vi "Single motor operation(Wheel mode).vi"() -> ()   [LabVIEW 2016]
uses:
  <instrlib>/Dynamixel Motor/Public/Motor Operation/Low Level/Baud Setting.ctl
  <instrlib>/Dynamixel Motor/Dynamixel Motor.lvlib
panel:
  in  "Goal Speed (RPM)":dbl
  in  "Motor ID (0)":u8
  in  "정지":bool
  in  "Baud rate (57600 bps)":T1=34 items=["1,000,000 bps"=1, "500,000 bps"=3, "400,000 bps"=4, "250,000 bps"=7, "200,000 bps"=9, "115200 bps"=16, "57600 bps"=34, "19200 bps"=103, "9600 bps"=207]
  in  "VISA resource name":refnum<visa-resource-name>
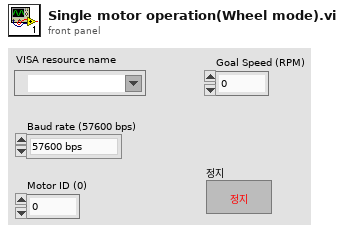
[diagram p1: front panel]
types:
  T1 = typedef "Dynamixel Motor.lvlib/Baud Setting.ctl" = u8
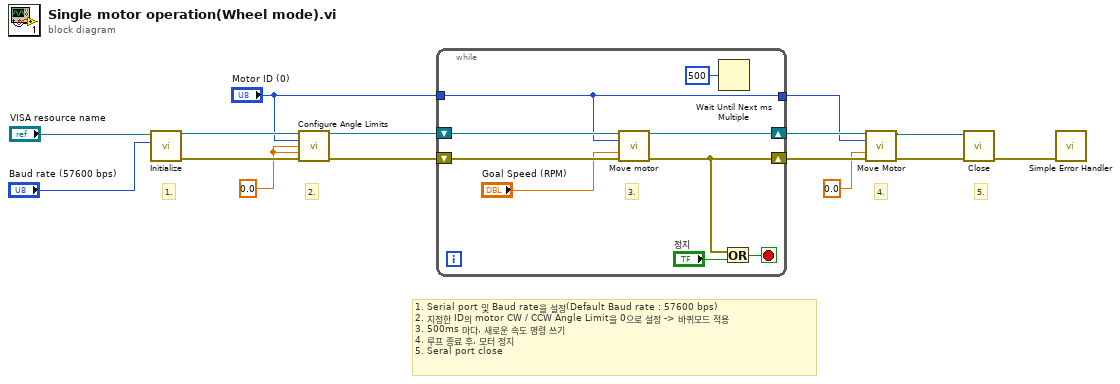
[diagram p0: block diagram]
diagram:
  w8 = 0.0 ("Clockwise Angle Limit (0 deg)")
  # "5."
  # "1. Serial port 및 Baud rate을 설정(Default Baud rate : 57600 bps)\n2. 지정한 ID의 motor CW / CCW Angle Limit을 0으로 설정 -> 바퀴모드 적용\n3. 500ms 마다, 새로운 속도 명령 쓰기\n4. 루프 종료 후, 모터 정지\n5. Seral port close"
  # "2."
  # "4."
  # "1."
  n1 = call <instrlib>:"Initialize.vi"("Baud rate (57600 bps)"="Baud rate (57600 bps)", "VISA resource name"="VISA resource name") -> ("error out"=w14:errorcluster, "VISA resource name out"=w15:refnum<visa-resource-name>)  [unwired: 8 in]
  n2 = call <instrlib>:"Configure Angle Limits.vi"("VISA resource name"=w15, "Motor ID (0)"="Motor ID (0)", "Clockwise Angle Limit (0 deg)"=w8, "Counter-Clockwise Angle Limit (300 deg)"=w8, "error in (no error)"=w14) -> ("VISA resource name out"=w10:refnum<visa-resource-name>, "error out"=w9:errorcluster)  [unwired: 9 in]
  n3 = while {
    shift-right: [w22] -> w5
    shift-left: w10 -> [w24]
    shift-right: [w17] -> w4
    shift-left: w9 -> [w23]
    tunnel: "Motor ID (0)" -> [w19]
    tunnel: [w19] -> w2
    stop <- w16 stop-if-true
    # "3."
    n4 = call <instrlib>:"Move motor.vi"("VISA resource name"=w24, "Motor ID (0)"=w19, "Goal Speed (RPM)"="Goal Speed (RPM)", "error in (no error)"=w23) -> ("VISA resource name out"=w22:refnum<visa-resource-name>, "error out"=w17:errorcluster)  [unwired: 10 in]
    n5 = Wait Until Next ms Multiple(millisecond multiple=u32 500 ("ms 배수")) -> ()  [unwired: 1 out]
    n6 = Or(x=w17, y="정지") -> (x .or. y?=w16:bool)
  }
  n7 = call <instrlib>:"Move Motor.vi"("VISA resource name"=w5, "Motor ID (0)"=w2, "Goal Speed (RPM)"=0.0, "error in (no error)"=w4) -> ("VISA resource name out"=w3:refnum<visa-resource-name>, "error out"=w6:errorcluster)  [unwired: 10 in]
  n8 = call <instrlib>:"Close.vi"("error in (no error)"=w6, "VISA resource name"=w3) -> ("error out"=w13:errorcluster)  [unwired: 9 in]
  n9 = call <vilib>:"Simple Error Handler.vi"("error in (no error)"=w13) -> ()  [unwired: 4 in, 5 out]
